vi "TestCloneAPI.vi"() -> ()   [LabVIEW 2018, in "SensorModule.lvlib"]
uses:
  SensorModule.lvlib
  TestInfo.ctl
  <userlib>/NIST/ModuleAdminLib/CloneRegistration/CloneRegistration.lvclass
  <userlib>/NIST/ModuleAdminLib/ModuleAdmin/ModuleAdmin.lvclass/ModuleAdmin.ctl
  <userlib>/NIST/ModuleAdminLib/ModuleAdmin/ModuleAdmin.lvclass
  PublicAPI/Arguments/Broadcasts/clDidInit.ctl
  PublicAPI/Arguments/Requests/clStopArgument.ctl
  <userlib>/NIST/ModuleAdminLib/ModuleAdmin/Accessors/Read CloneRegRef.vi
  <userlib>/NIST/ModuleAdminLib/ModuleAdmin/Accessors/Write CloneRegRef.vi
  SensorPlugins/SensorBaseClass/SensorBase.lvclass
panel:
  in  "btnConfigure":bool
  in  "btnStopData":bool
  in  "btnStartData":bool
  in  "Show Panel":bool=TRUE
  in  "Plugin Type":u16(ring) items=["C37.118 PMU", "C37.118 Sim", "Base PMU", "Base Plugin"]
  in  "btnLoadPlugin":bool
  out "Path":path
  in  "btnRequestINIPath":bool
  in  "btnRemove":bool
  out "Status Log":string
  out "Active Modules (Array)":string[](array[string])
  in  "btnAdd":bool
  in  "btnStop":bool
  in  "Select Module":i32(ring)=-1 caption="Select Module to send Request" items=["All"=-1, "4140003"=4140003]
  # "Hidden"
  # "Visible"
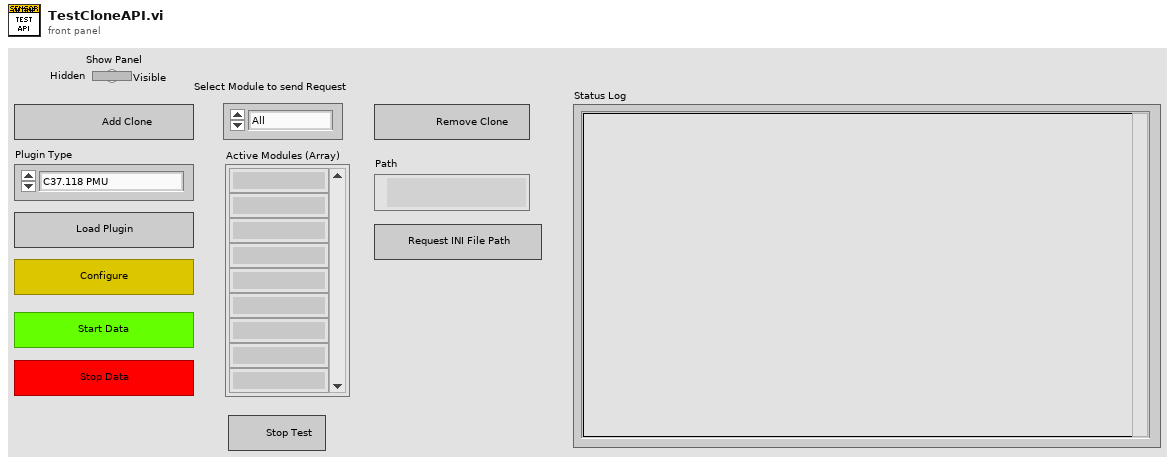
[diagram p1: front panel]
types:
  T1 = typedef "SensorModule.lvlib/TestInfo.ctl" = cluster{"PluginIniFilePaths":path[]}
  T2 = typedef "SensorModule.lvlib/clBroadcastEvents.ctl" = cluster{"DidInit":refnum<user-event>, "StatusUpdate":refnum<user-event>, "ErrorReport":refnum<user-event>, "DidStop":refnum<user-event>, "PathToINI":refnum<user-event>, "SensorReport":refnum<user-event>, "SensorConfig":refnum<user-event>}
  T3 = typedef "SensorModule.lvlib/clDidInit.ctl" = cluster{"Init?":bool, "ModuleAdmin":refnum<class "ModuleAdmin.lvclass">}
  T4 = typedef "SensorModule.lvlib/clStopArgument.ctl" = cluster{"Exit via Stop Module Req?":bool, "Wait for Module to stop?":bool, "ModuleAdmin":refnum<class "ModuleAdmin.lvclass">}
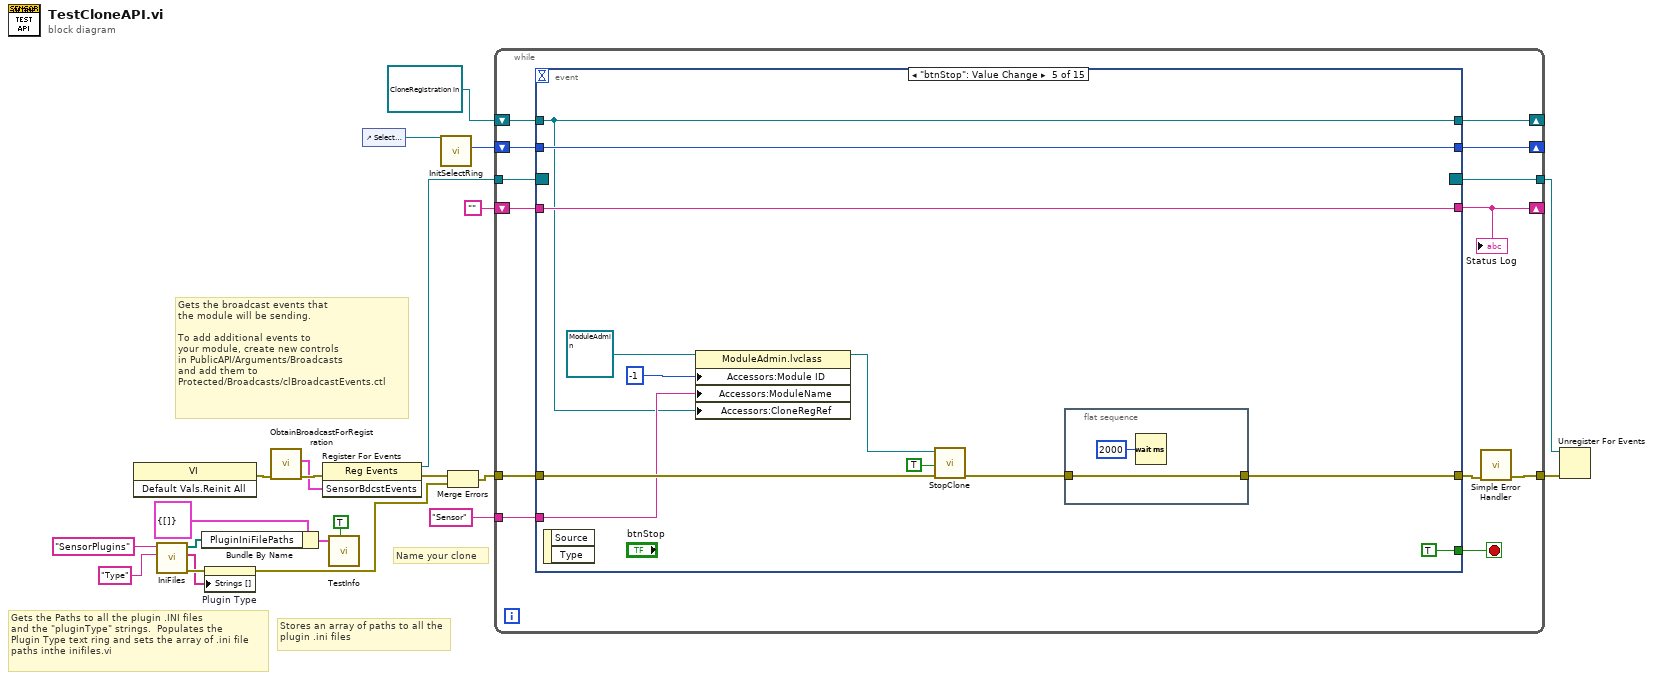
[diagram p0: block diagram]
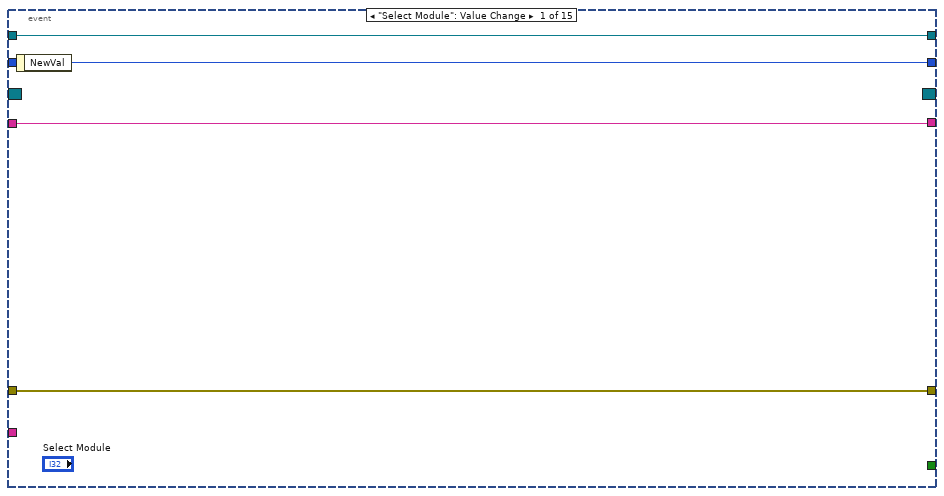
[diagram p2: hidden frame]
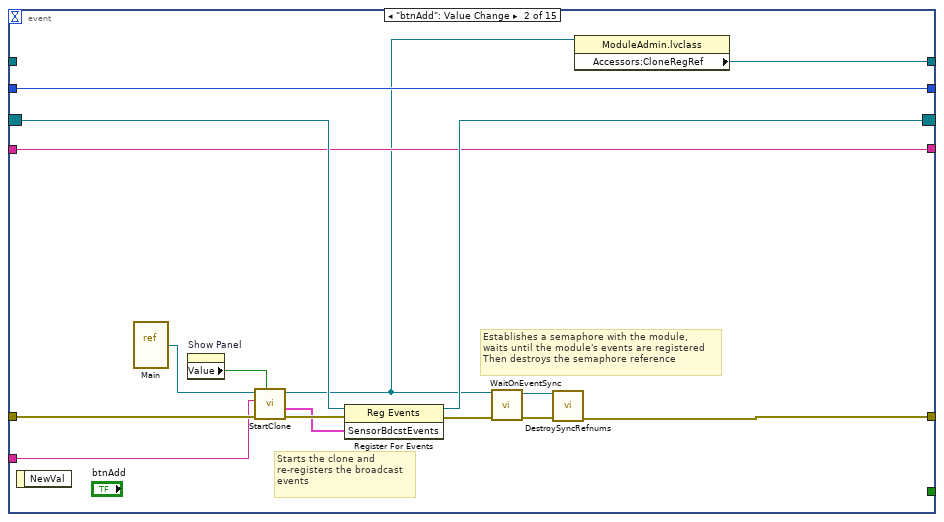
[diagram p3: hidden frame]
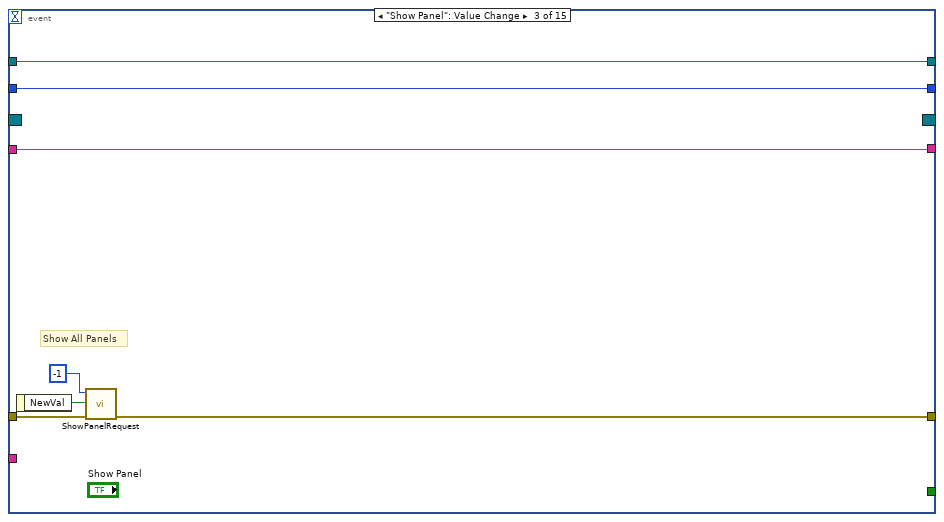
[diagram p4: hidden frame]
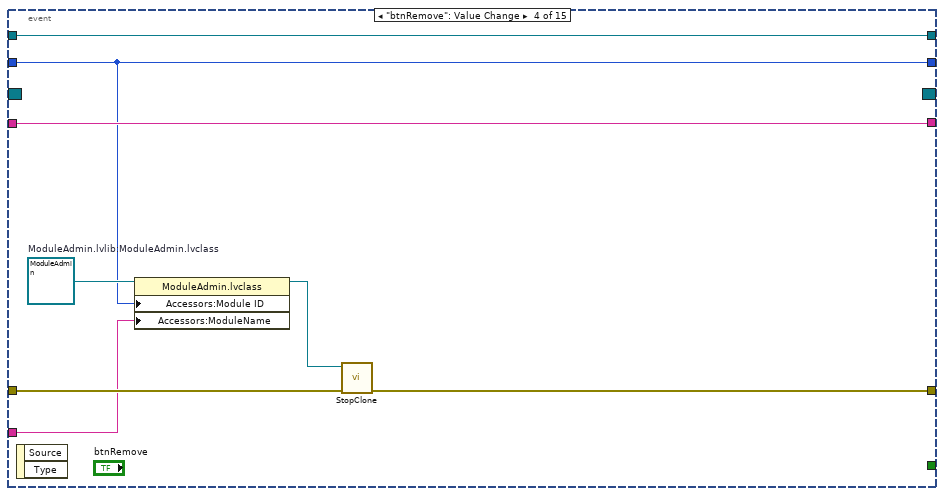
[diagram p5: hidden frame]
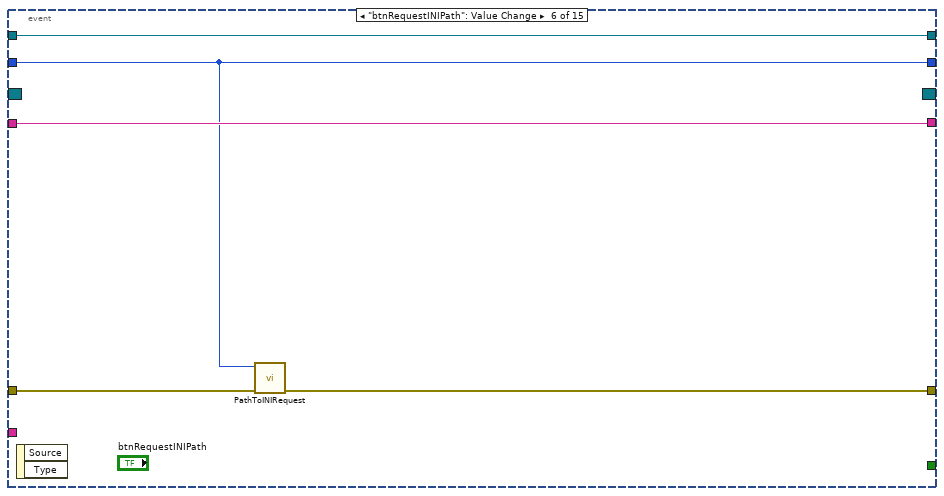
[diagram p6: hidden frame]
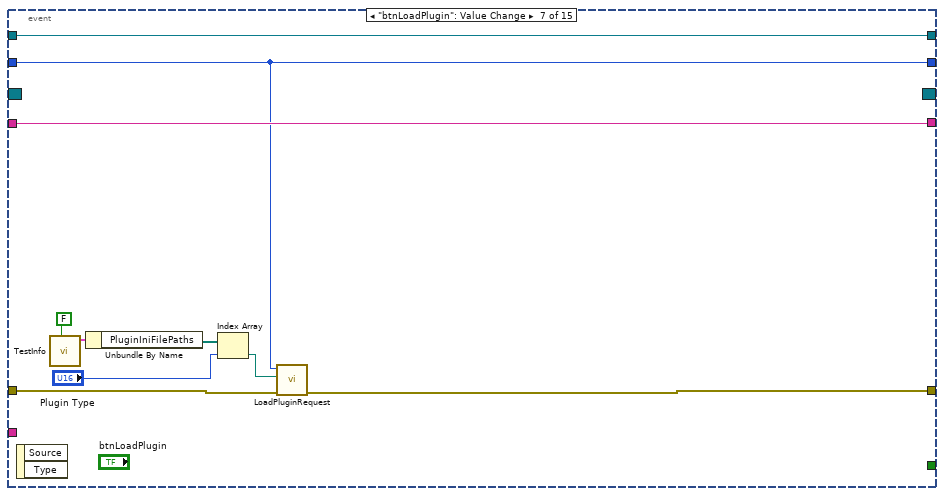
[diagram p7: hidden frame]
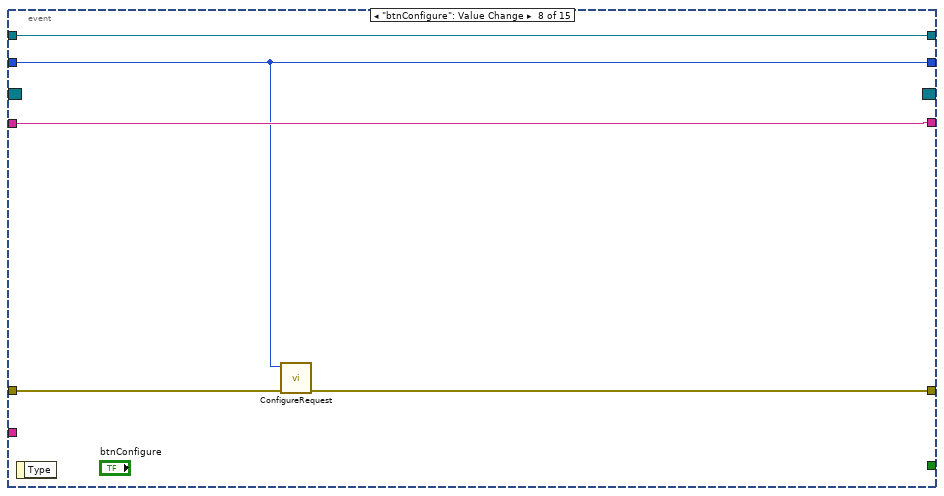
[diagram p8: hidden frame]
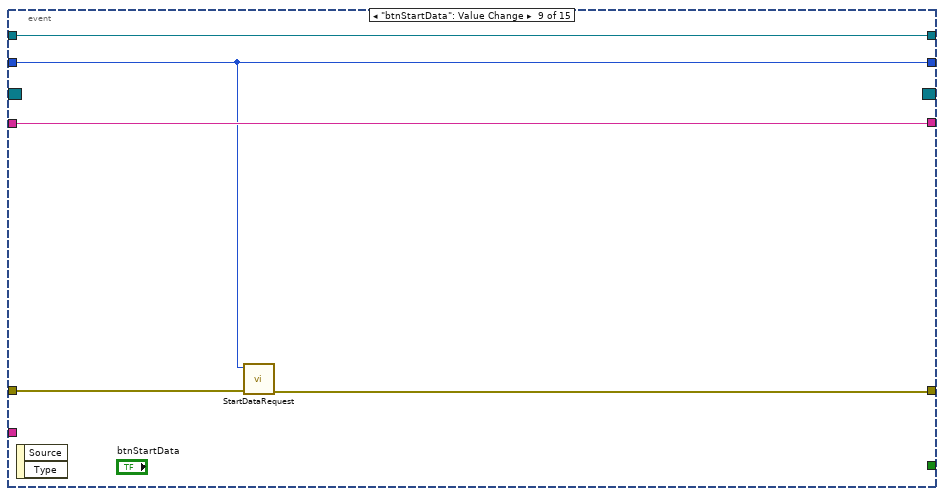
[diagram p9: hidden frame]
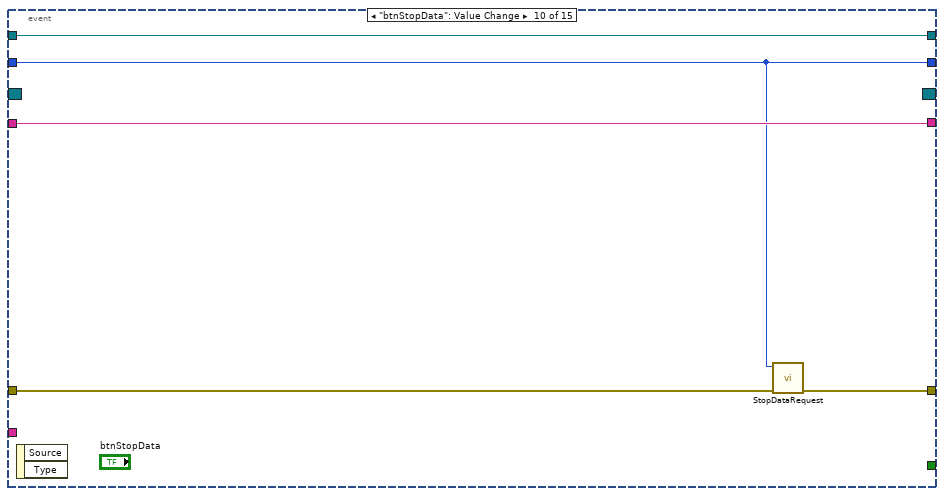
[diagram p10: hidden frame]
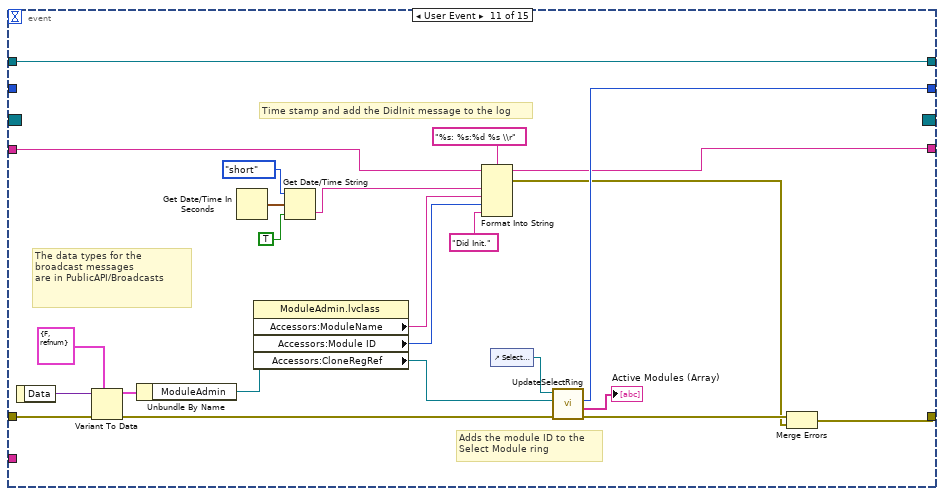
[diagram p11: hidden frame]
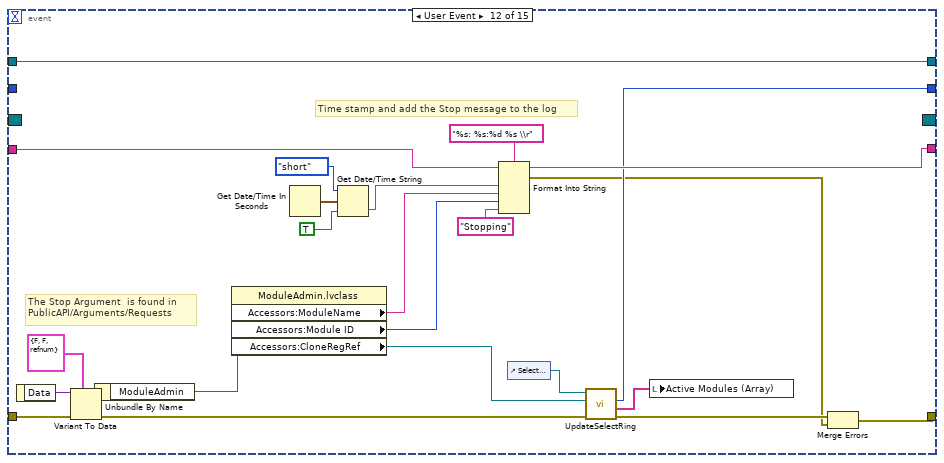
[diagram p12: hidden frame]
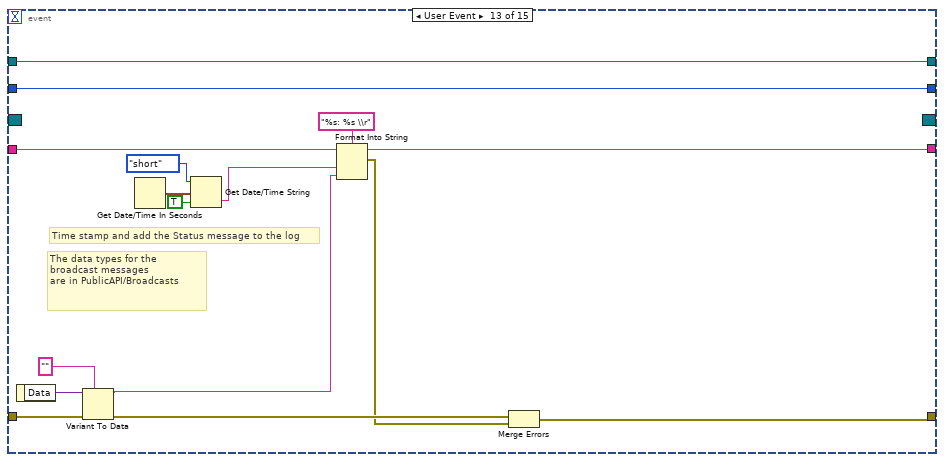
[diagram p13: hidden frame]
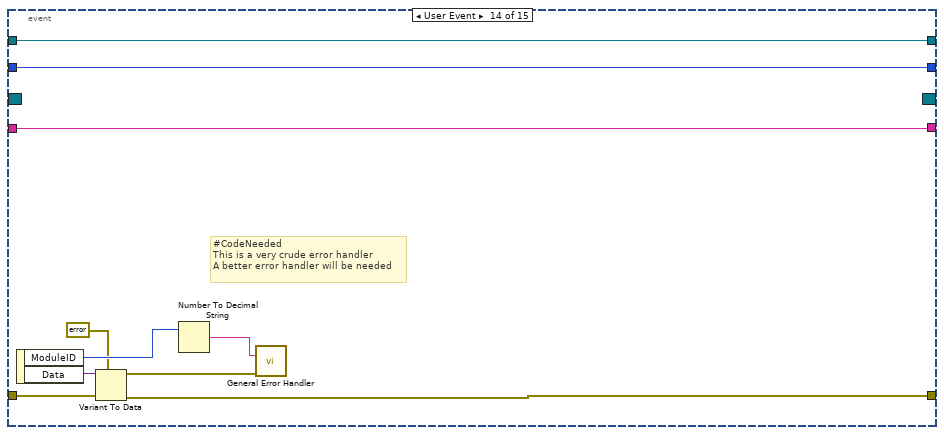
[diagram p14: hidden frame]
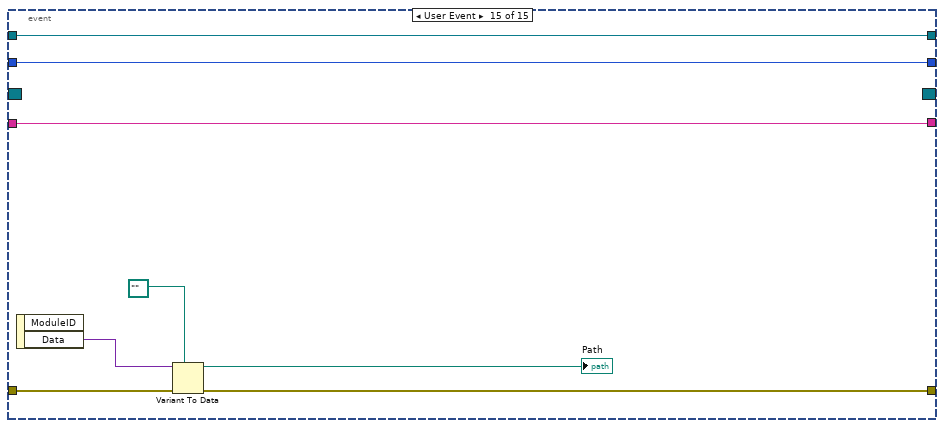
[diagram p15: hidden frame]
diagram:
  # "Stores an array of paths to all the plugin .ini files"
  # "Gets the Paths to all the plugin .INI files\nand the \"pluginType\" strings.  Populates the \nPlugin Type text ring and sets the array of .ini file\npaths inthe inifiles.vi"
  # "Name your clone"
  # "Gets the broadcast events that\nthe module will be sending.\n\nTo add additional events to\nyour module, create new controls\nin PublicAPI/Arguments/Broadcasts\nand add them to\nProtected/Broadcasts/clBroadcastEvents.ctl"
  n1 = invoke class="VI" method="Default Vals.Reinit All"() -> (error out=w20:errorcluster)  [unwired: 3 in, 2 out]
  n2 = call "IniFiles.vi"("iniKey"="Type", "name or relative path"="SensorPlugins") -> ("error out"=w13:errorcluster, "Types"=w12:string[], "IniFilePaths"=w11:path[])  [unwired: 7 in]
  n3 = Bundle By Name(cluster=T1 {"PluginIniFilePaths"=[]} ("TestInfo"), "PluginIniFilePaths"=w11) -> (w10:T1)
  n4 = property on="Plugin Type" class="Ring (strict)"(error in=w13, "Strings []"=w12) -> (error out=w7:errorcluster)  [unwired: 1 in, 1 out]
  n5 = call "ObtainBroadcastForRegistration.vi"("error in (no error)"=w20) -> ("error out"=w19:errorcluster, "SensorBdcstEvents"=w18:T2)  [unwired: 9 in]
  n6 = register-events(error in=w19, w18) -> (reference out=w16:refnum<event-registration>, error out=w17:errorcluster)  [unwired: 1 in]
  n7 = call "TestInfo.vi"("Set (f)"=TRUE, "TestInfo 2"=w10) -> ()  [unwired: 9 in, 1 out]
  n8 = control-ref of="Select Module"() -> (w22:refnum<vi>)
  n9 = call "InitSelectRing.vi"("Ring Refnum"=w22) -> ("Module Ring Value"=w21:i32)  [unwired: 9 in, 1 out]
  n10 = Merge Errors(w17, w7) -> (w8:errorcluster)
  n11 = while {
    shift-right: [w34] -> _
    shift-left: w21 -> [w35]
    tunnel: w8 -> [w32]
    tunnel: w16 -> [w29]
    tunnel: [w30] -> w3
    shift-right: [w28] -> _
    shift-left: "" -> [w27]
    tunnel: "Sensor" ("ModuleName") -> [w26]
    tunnel: [w25] -> w2
    shift-right: [w24] -> _
    shift-left: refnum<data-value> refnum ("Accessors:CloneRegRef") -> [w23]
    stop <- w33 stop-if-true
    n12 = event shown="[4] \"btnStop\": Value Change" {
      selector: w29 -> [_ w47 _ _ _ _ _ _ _ _ _ _ _ _ _]
      dyn-events: [_ w46 _ _ _ _ _ _ _ _ _ _ _ _ _] -> w25
      timeout: _ -> [_ _ _ _ _ _ _ _ _ _ _ _ _ _ _]
      tunnel: w35 -> [_ w55 w58 w66 w82 w88 w96 w103 w106 w111 _ _ w178 w183 w195]
      tunnel: [w39 w55 w58 w66 w82 w88 w96 w103 w106 w111 w133 w149 w178 w183 w195] -> w34
      tunnel: [_ _ _ _ TRUE _ _ _ _ _ _ _ _ _ _] -> w33
      tunnel: w32 -> [w37 w54 w61 w69 w80 w87 w98 w102 w108 w113 w138 w158 w175 w187 w191]
      tunnel: [w37 w48 w59 w68 w72 w86 w97 w101 w107 w112 w122 w146 w169 w186 w190] -> w31
      tunnel: [w38 w44 w57 w70 w78 w89 w99 w104 w109 w114 w126 w155 w172 w182 w196] -> w28
      tunnel: w27 -> [w38 w44 w57 w70 w78 w89 w99 w104 w109 w114 w125 w156 w177 w182 w196]
      tunnel: w26 -> [_ w43 _ w65 w75 _ _ _ _ _ _ _ _ _ _]
      tunnel: [w36 w40 w56 w63 w73 w85 w90 w100 w105 w110 w115 w139 w163 w179 w189] -> w24
      tunnel: w23 -> [w36 _ w56 w63 w73 w85 w90 w100 w105 w110 w115 w139 w163 w179 w189]
      event "Select Module": Value Change {
        n13 = event-data() -> ("NewVal"=w39:i32)  [unwired: 1 in]
      }
      event "btnAdd": Value Change {
        # "Establishes a semaphore with the module,\nwaits until the module's events are registered\nThen destroys the semaphore reference"
        # "Starts the clone and\nre-registers the broadcast \nevents"
        n14 = event-data() -> ()  [unwired: 1 in, 1 out]
        n15 = vi-ref "Main.vi"() -> (w45:refnum<vi>)
        n16 = property on="Show Panel" class="Bool (strict)"() -> ("Value"=w42:bool)  [unwired: 2 in, 2 out]
        n17 = call "StartClone.vi"("ShowPanel? (f)"=w42, "error in (no error)"=w54, "ModuleName"=w43, "VI Refnum"=w45) -> ("error out"=w53:errorcluster, "clBroadcastEvents"=w49:T2, "ModuleAdmin"=w41:refnum<class "ModuleAdmin.lvclass">)  [unwired: 5 in]
        n18 = register-events(reference=w47, error in=w53, w49) -> (reference out=w46:refnum<event-registration>, error out=w52:errorcluster)
        n19 = call <userlib>:"WaitOnEventSync.vi"("error in (no error)"=w52, "ModuleAdmin"=w41) -> ("error out"=w51:errorcluster, "ModuleAdmin"=w50:refnum<class "ModuleAdmin.lvclass">)  [unwired: 8 in]
        n20 = call <userlib>:"DestroySyncRefnums.vi"("error in (no error)"=w51, "ModuleAdmin"=w50) -> ("error out"=w48:errorcluster)  [unwired: 9 in]
        n21 = property class="ModuleAdmin.lvclass"(reference=w41) -> ("Accessors:CloneRegRef"=w40:refnum<data-value>)  [unwired: 1 in, 2 out]
      }
      event "Show Panel": Value Change {
        # "Show All Panels"
        n22 = event-data() -> ("NewVal"=w62:bool)  [unwired: 1 in]
        n23 = call "ShowPanelRequest.vi"("error in (no error)"=w61, "ShowPanel?"=w62, "ModuleID"=-1) -> ("error out"=w59:errorcluster)  [unwired: 8 in]
      }
      event "btnRemove": Value Change {
        w67 = refnum<class "ModuleAdmin.lvclass"> refnum  # ModuleAdmin.lvlib:ModuleAdmin.lvclass
        n24 = event-data() -> ()  [unwired: 1 in, 2 out]
        n25 = property class="ModuleAdmin.lvclass"(reference=w67, "Accessors:Module ID"=w66, "Accessors:ModuleName"=w65) -> (reference out=w64:refnum<class "ModuleAdmin.lvclass">)  [unwired: 1 in, 1 out]
        n26 = call "StopClone.vi"("error in (no error)"=w69, "ModuleAdmin"=w64) -> ("error out"=w68:errorcluster)  [unwired: 9 in]
      }
      event "btnStop": Value Change {
        n27 = event-data() -> ()  [unwired: 1 in, 2 out]
        n28 = property class="ModuleAdmin.lvclass"(reference=refnum<class "ModuleAdmin.lvclass"> refnum ("ModuleAdmin.lvlib:ModuleAdmin.lvclass"), "Accessors:Module ID"=-1 ("Module ID"), "Accessors:ModuleName"=w75, "Accessors:CloneRegRef"=w73) -> (reference out=w74:refnum<class "ModuleAdmin.lvclass">)  [unwired: 1 in, 1 out]
        n29 = call "StopClone.vi"("error in (no error)"=w80, "Wait for Module to stop?"=TRUE, "ModuleAdmin"=w74) -> ("error out"=w71:errorcluster)  [unwired: 8 in]
        n30 = flat-sequence {
          tunnel: [w83] -> w72
          tunnel: w71 -> [w83]
          frame #0 {
            n31 = Wait (ms)(milliseconds to wait=u32 2000) -> ()  [unwired: 1 out]
          }
        }
      }
      event "btnRequestINIPath": Value Change {
        n32 = event-data() -> ()  [unwired: 1 in, 2 out]
        n33 = call "PathToINIRequest.vi"("error in (no error)"=w87, "ModuleID"=w88) -> ("error out"=w86:errorcluster)  [unwired: 9 in]
      }
      event "btnLoadPlugin": Value Change {
        n34 = event-data() -> ()  [unwired: 1 in, 2 out]
        n35 = call "TestInfo.vi"("Set (f)"=FALSE) -> ("TestInfo"=w94:T1)  [unwired: 10 in]
        n36 = Unbundle By Name(w94) -> ("PluginIniFilePaths"=w93:path[])
        n37 = Index Array(array=w93, index="Plugin Type") -> (element=w91:path)
        n38 = call "LoadPluginRequest.vi"("error in (no error)"=w98, "PathToPluginINI"=w91, "ModuleID"=w96) -> ("error out"=w97:errorcluster)  [unwired: 8 in]
      }
      event "btnConfigure": Value Change {
        n39 = event-data() -> ()  [unwired: 1 in, 1 out]
        n40 = call "ConfigureRequest.vi"("error in (no error)"=w102, "ModuleID"=w103) -> ("error out"=w101:errorcluster)  [unwired: 9 in]
      }
      event "btnStartData": Value Change {
        n41 = event-data() -> ()  [unwired: 1 in, 2 out]
        n42 = call "StartDataRequest.vi"("error in (no error)"=w108, "ModuleID"=w106) -> ("error out"=w107:errorcluster)  [unwired: 9 in]
      }
      event "btnStopData": Value Change {
        n43 = event-data() -> ()  [unwired: 1 in, 2 out]
        n44 = call "StopDataRequest.vi"("error in (no error)"=w113, "ModuleID"=w111) -> ("error out"=w112:errorcluster)  [unwired: 9 in]
      }
      event User Event {
        # "Adds the module ID to the \nSelect Module ring"
        # "Time stamp and add the DidInit message to the log"
        # "The data types for the broadcast messages\nare in PublicAPI/Broadcasts"
        n45 = event-data() -> ("Data"=w137:variant)  [unwired: 1 in]
        n46 = Variant To Data(error in=w138, type=T3 {"Init?"=FALSE, "ModuleAdmin"=refnum} ("clDidInit"), Variant=w137) -> (data=w130:T3, error out=w135:errorcluster)
        n47 = Unbundle By Name(w130) -> ("ModuleAdmin"=w120:refnum<class "ModuleAdmin.lvclass">)
        n48 = Get Date/Time In Seconds() -> (seconds since 1Jan1904=w128:timestamp)
        n49 = property class="ModuleAdmin.lvclass"(reference=w120) -> ("Accessors:ModuleName"=w118:string, "Accessors:Module ID"=w117:i32, "Accessors:CloneRegRef"=w116:refnum<data-value>)  [unwired: 1 in, 2 out]
        n50 = Get Date/Time String(date format (0)=enum16{"short", "long", "abbreviated"}."short", seconds (now)=w128, want seconds? (F)=TRUE) -> (time string=w131:string)  [unwired: 1 out]
        n51 = Format Into String(format string="%s: %s:%d %s \\r", initial string=w125, w131, w118, w117, "Did Init.") -> (resulting string=w126:string, error out=w123:errorcluster)  [unwired: 1 in]
        n52 = control-ref of="Select Module"() -> (w134:refnum<vi>)
        n53 = call "UpdateSelectRing.vi"("error in (no error)"=w135, "CloneRegRef"=w116, "Ring Refnum"=w134) -> ("error out"=w124:errorcluster, "ActiveModules"=→"Active Modules (Array)":string[], "Module Ring Value"=w133:i32)  [unwired: 6 in]
        n54 = Merge Errors(w124, w123) -> (w122:errorcluster)
      }
      event User Event {
        # "Time stamp and add the Stop message to the log"
        # "The Stop Argument  is found in\nPublicAPI/Arguments/Requests"
        n55 = event-data() -> ("Data"=w157:variant)  [unwired: 1 in]
        n56 = Variant To Data(error in=w158, type=T4 {"Exit via Stop Module Req?"=FALSE, "Wait for Module to stop?"=FALSE, "ModuleAdmin"=refnum} ("Stop Argument"), Variant=w157) -> (data=w153:T4, error out=w152:errorcluster)
        n57 = Unbundle By Name(w153) -> ("ModuleAdmin"=w144:refnum<class "ModuleAdmin.lvclass">)
        n58 = property class="ModuleAdmin.lvclass"(reference=w144) -> ("Accessors:ModuleName"=w142:string, "Accessors:Module ID"=w141:i32, "Accessors:CloneRegRef"=w140:refnum<data-value>)  [unwired: 1 in, 2 out]
        n59 = Get Date/Time In Seconds() -> (seconds since 1Jan1904=w160:timestamp)
        n60 = Get Date/Time String(date format (0)=enum16{"short", "long", "abbreviated"}."short", seconds (now)=w160, want seconds? (F)=TRUE) -> (time string=w162:string)  [unwired: 1 out]
        n61 = Format Into String(format string="%s: %s:%d %s \\r", initial string=w156, w162, w142, w141, "Stopping") -> (resulting string=w155:string, error out=w147:errorcluster)  [unwired: 1 in]
        n62 = control-ref of="Select Module"() -> (w151:refnum<vi>)
        n63 = call "UpdateSelectRing.vi"("error in (no error)"=w152, "CloneRegRef"=w140, "Ring Refnum"=w151) -> ("error out"=w148:errorcluster, "ActiveModules"=w150:string[], "Module Ring Value"=w149:i32)  [unwired: 6 in]
        n64 = local write "Active Modules (Array)"(w150) -> ()
        n65 = Merge Errors(w148, w147) -> (w146:errorcluster)
      }
      event User Event {
        # "Time stamp and add the Status message to the log"
        # "The data types for the broadcast messages\nare in PublicAPI/Broadcasts"
        n66 = event-data() -> ("Data"=w174:variant)  [unwired: 1 in]
        n67 = Variant To Data(error in=w175, type="", Variant=w174) -> (data=w164:string, error out=w171:errorcluster)
        n68 = Get Date/Time In Seconds() -> (seconds since 1Jan1904=w173:timestamp)
        n69 = Get Date/Time String(date format (0)=enum16{"short", "long", "abbreviated"}."short", seconds (now)=w173, want seconds? (F)=TRUE) -> (time string=w166:string)  [unwired: 1 out]
        n70 = Format Into String(format string="%s: %s \\r", initial string=w177, w166, w164) -> (resulting string=w172:string, error out=w170:errorcluster)  [unwired: 1 in]
        n71 = Merge Errors(w171, w170) -> (w169:errorcluster)
      }
      event User Event {
        # "#CodeNeeded\nThis is a very crude error handler\nA better error handler will be needed"
        n72 = event-data() -> ("ModuleID"=w185:i32, "Data"=w188:variant)  [unwired: 1 in]
        n73 = Variant To Data(error in=w187, type=errorcluster {"status"=FALSE, "code"=0, "source"=""} ("error constant"), Variant=w188) -> (data=w180:errorcluster, error out=w186:errorcluster)
        n74 = Number To Decimal String(number=w185) -> (decimal integer string=w184:string)  [unwired: 1 in]
        n75 = call <vilib>:"General Error Handler.vi"("[error source] (\" \")"=w184, "error in (no error)"=w180) -> ()  [unwired: 9 in, 5 out]
      }
      event User Event {
        n76 = event-data() -> ("Data"=w193:variant)  [unwired: 1 in, 1 out]
        n77 = Variant To Data(error in=w191, type=path "" ("Path"), Variant=w193) -> (data=→"Path":path, error out=w190:errorcluster)
      }
    }
    "Status Log" <- w28
    n78 = call <vilib>:"Simple Error Handler.vi"("error in (no error)"=w31) -> ("error out"=w30:errorcluster)  [unwired: 4 in, 4 out]
  }
  n79 = Unregister For Events(event registration refnum=w2, error in=w3) -> ()  [unwired: 1 out]
